vi "MakeDataFileForMultiplot.vi"(0 "Legend":string[](array[string]), 1 "Path":path, 3 "Plot Array":cluster{"Angle":dbl[], "Radius":dbl[]}[](array[cluster]), 5 "Plot Summary":string[][](array[string]), 9 "Transpose":bool, 11 "Error Bar Cluster":T2[](array[typedef]), 12 "X Axis Name":string, 13 "Y Axis Name":string, 14 "Error Bar Type":T1) -> ()   [LabVIEW 2016]
uses:
  Error_bars.ctl
  Error bar Type.ctl
  Results_plotter_Global.vi
panel:
  out "datLoops":i32
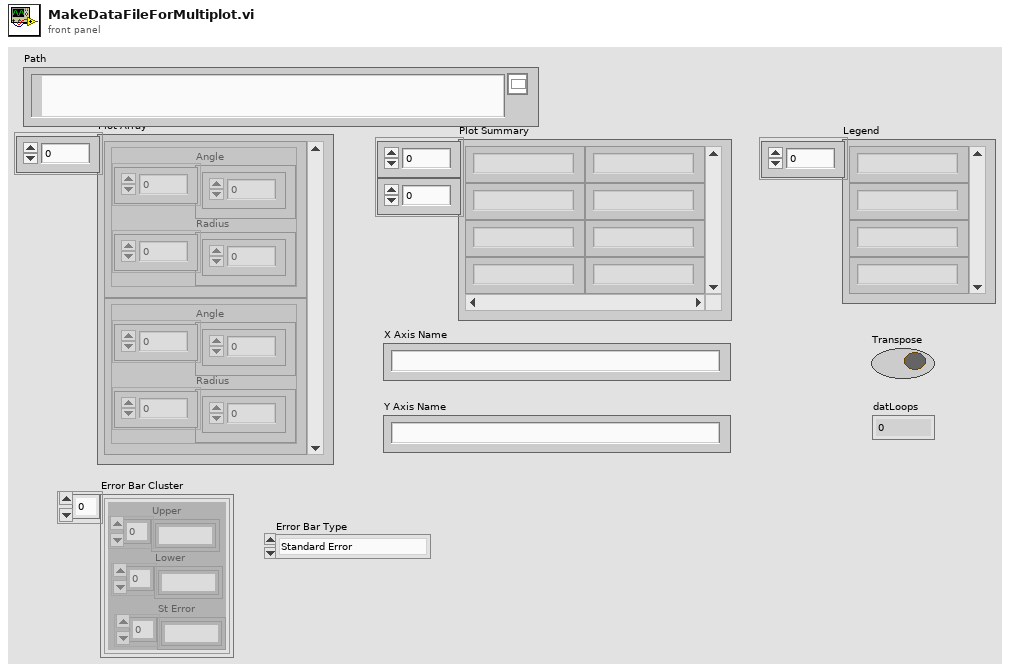
[diagram p1: front panel]
types:
  T1 = typedef "Error bar Type.ctl" = enum16{"Standard Error", "Separate upper and lower"}
  T2 = typedef "Error_bars.ctl" = cluster{"Upper":string[], "Lower":string[], "St Error":string[]}
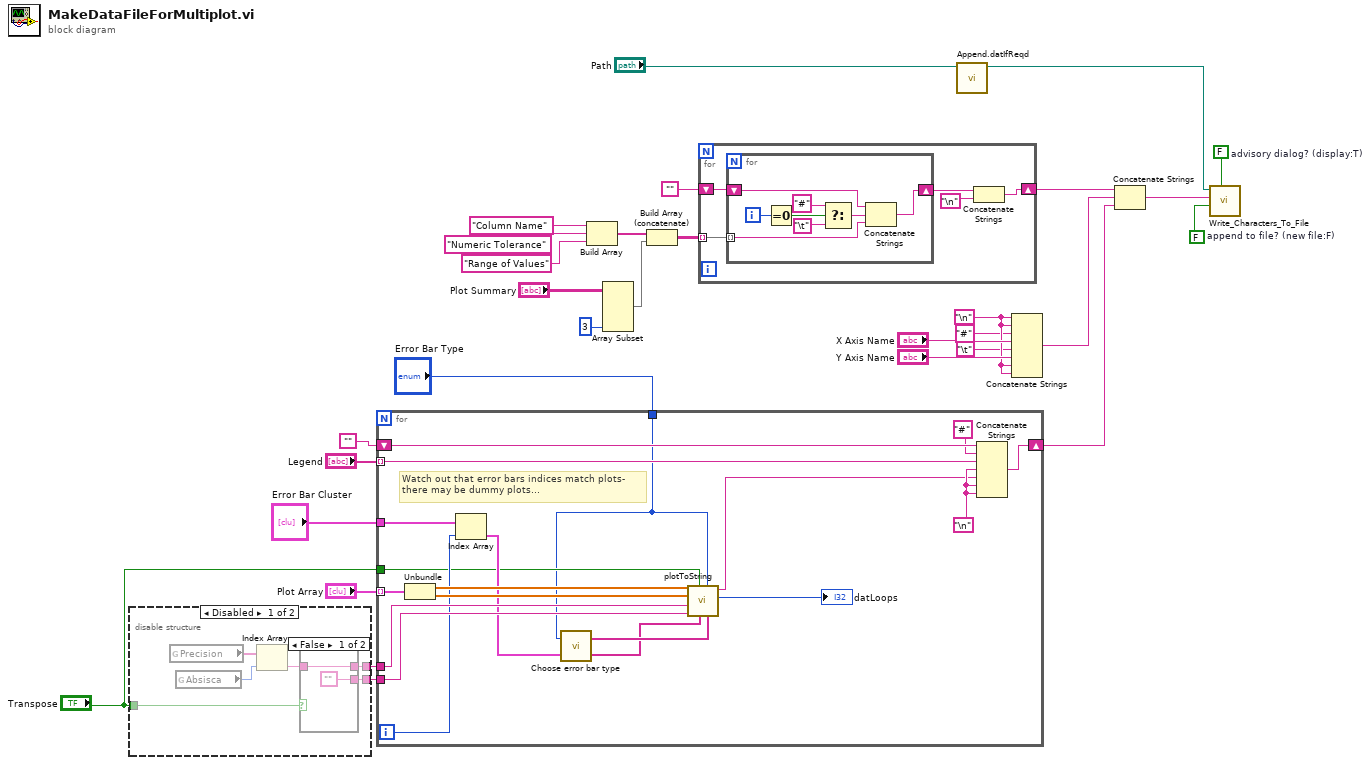
[diagram p0: block diagram]
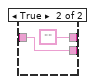
[diagram p2: hidden frame]
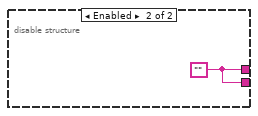
[diagram p3: hidden frame]
diagram:
  w10 = FALSE  # advisory dialog? (display:T)
  w9 = FALSE  # append to file? (new file:F)
  w19 = "\n"
  n1 = disable-structure shown="Disabled" {
    disable-tunnel: [w33 w41] -> w13
    disable-tunnel: [w32 w41] -> w12
    disable-tunnel: "Transpose" -> [w31 _]
    frame Disabled {
      n2 = global read "Results_plotter_Global.vi" "Precision"() -> (w34:string[])
      n3 = global read "Results_plotter_Global.vi" "Absisca"() -> (w35:i32)
      n4 = Index Array(array=w34, index=w35) -> (element=w36:string)
      n5 = case shown="False" w31 {
        tunnel: ["" w40] -> w32
        tunnel: w36 -> [w37 w40]
        tunnel: [w37 ""] -> w33
        frame False {
        }
        frame True {
        }
      }
    }
    frame Enabled {
      w41 = ""
    }
  }
  n6 = for {
    tunnel: "Plot Array" -> [w60] mode=indexing
    shift-right: [w59] -> w5
    shift-left: "" -> [w54]
    tunnel: "Legend" -> [w52] mode=indexing
    tunnel: w13 -> [w51]
    tunnel: w12 -> [w49]
    tunnel: "Error Bar Cluster" -> [w48]
    tunnel: "Error Bar Type" -> [w42]
    tunnel: "Transpose" -> [w43]
    i -> [w47]
    w58 = "\n"
    # "Watch out that error bars indices match plots-\nthere may be dummy plots..."
    n7 = Unbundle(w60) -> ("Angle"=w55:dbl[], "Radius"=w56:dbl[])
    n8 = Index Array(array=w48, index=w47) -> (element=w46:T2)
    n9 = call "Choose error bar type.vi"("Error_bars"=w46, "Error Bar Type"=w42) -> ("Lower"=w44:string[], "Upper"=w45:string[])
    n10 = call "plotToString.vi"("Error Bar upper"=w45, "Error Bar Type"=w42, "Error Bar lower"=w44, "Transpose"=w43, "Precision2"=w49, "Precision1"=w51, "Column2"=w56, "Column1"=w55) -> ("nLoops"=→"datLoops":i32, "plotString"=w57:string)  [unwired: 2 in]
    n11 = Concatenate Strings(w54, "#", w52, w58, w57, w58, w58) -> (w59:string)
  }
  n12 = Build Array("Column Name", "Numeric Tolerance", "Range of Values") -> (w22:string[])
  n13 = Array Subset(array="Plot Summary", length (col)=3 ("length")) -> (w27:string[][])  [unwired: 3 in]
  n14 = Build Array (concatenate)(w22, w27) -> (w29:string[][])
  n15 = for {
    shift-right: [w64] -> w7
    shift-left: "" -> [w61]
    tunnel: w29 -> [w65] mode=indexing
    n16 = for {
      shift-right: [w66] -> w63
      shift-left: w61 -> [w73]
      tunnel: w65 -> [w67] mode=indexing
      i -> [w72]
      n17 = Equal To 0?(x=w72) -> (x = 0?=w71:bool)
      n18 = Select(t="#", s=w71, f="\t") -> (s? t:f=w68:string)
      n19 = Concatenate Strings(w73, w68, w67) -> (w66:string)
    }
    n20 = Concatenate Strings(w63, "\n") -> (w64:string)
  }
  n21 = call "Append.datIfReqd.vi"("Path"="Path") -> ("appended path"=w11:path)  [unwired: 10 in]
  n22 = Concatenate Strings(w19, w19, "#" ("string"), "X Axis Name", "\t", "Y Axis Name", w19, w19) -> (w6:string)
  n23 = Concatenate Strings(w7, w6, w5) -> (w8:string)
  n24 = call "Write_Characters_To_File.vi"("file path (dialog if empty)"=w11, "advisory dialog? (display:T)"=w10, "character string"=w8, "append to file? (new file:F)"=w9) -> ()  [unwired: 1 in, 4 out]
